vi "QueueDriver.vi"(0 "Queue Name":string, 5 "State & Data":T1, 7 "Array of States & Data":T1[](array[typedef]), 11 "Error in (no error)":errorcluster, 13 "Operations":T2) -> (4 "Dequeued State & Variant":T1, 15 "Error out":errorcluster)   [LabVIEW 2020]
uses:
  Typedef/QueueOperation.ctl
  Typedef/State & Varaint.ctl
panel:
  # "Queue Driver"
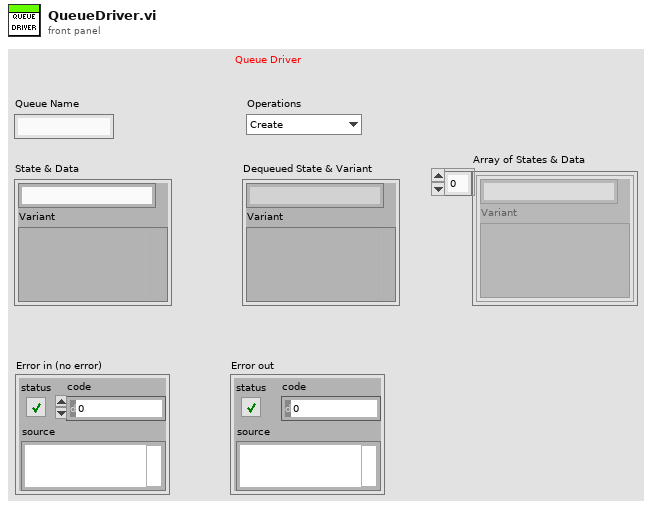
[diagram p1: front panel]
types:
  T1 = typedef "State & Varaint.ctl" = cluster{"State":string, "Variant":variant}
  T2 = typedef "QueueOperation.ctl" = enum16{"Create", "Enqueue 1", "Enqueue N", "Enstack 1", "Enstack N", "Dequeue", "Flush", "Release"}
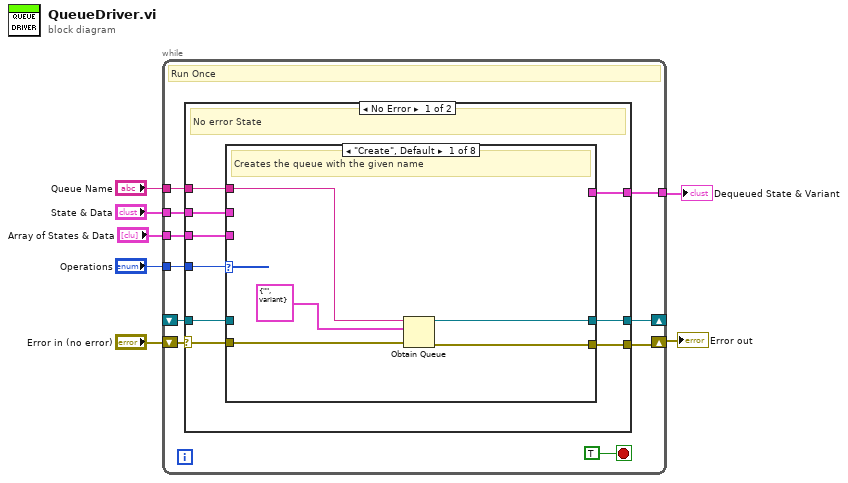
[diagram p0: block diagram]
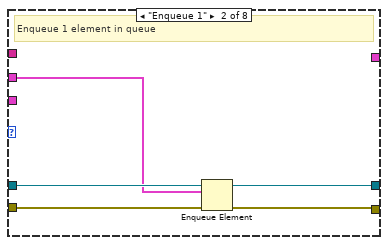
[diagram p2: hidden frame]
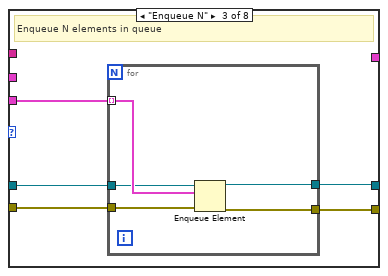
[diagram p3: hidden frame]
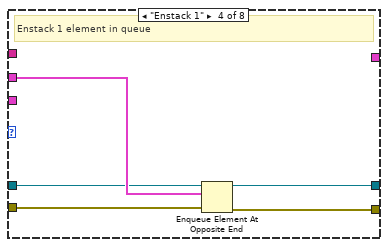
[diagram p4: hidden frame]
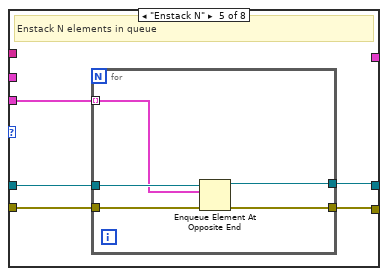
[diagram p5: hidden frame]
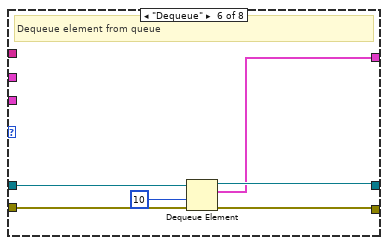
[diagram p6: hidden frame]
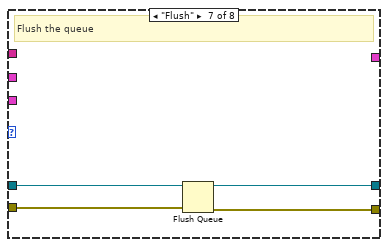
[diagram p7: hidden frame]
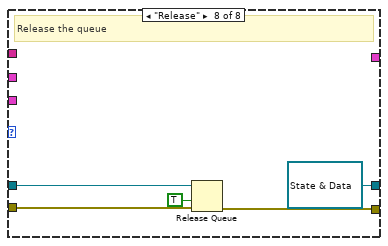
[diagram p8: hidden frame]
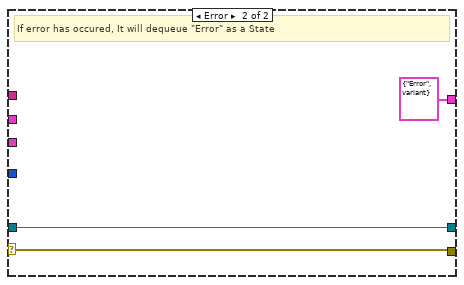
[diagram p9: hidden frame]
diagram:
  n1 = while {
    tunnel: "Operations" -> [w17]
    tunnel: "Queue Name" -> [w14]
    shift-right: [w9] -> _
    shift-left: _ -> [w12]
    tunnel: "State & Data" -> [w11]
    tunnel: "Array of States & Data" -> [w10]
    tunnel: [w8] -> w1
    shift-right: [w13] -> w4
    shift-left: "Error in (no error)" -> [w15]
    stop <- TRUE stop-if-true
    # "Run Once"
    n2 = case shown="No Error" w15 {
      selector: w15 -> [w25 w77]
      tunnel: w17 -> [w26 _]
      tunnel: w14 -> [w24 _]
      tunnel: [w23 w77] -> w13
      tunnel: w12 -> [w22 w78]
      tunnel: w11 -> [w21 _]
      tunnel: w10 -> [w20 _]
      tunnel: [w19 w78] -> w9
      tunnel: [w18 T1 {"State"="Error", "Variant"=variant} ("State & Data")] -> w8
      frame No Error {
        # "No error State"
        n3 = case shown="\"Create\", Default" w26 {
          tunnel: w25 -> [w31 w36 w41 w51 w56 w67 w71 w76]
          tunnel: w24 -> [w30 _ _ _ _ _ _ _]
          tunnel: [w29 w35 w40 w50 w55 w66 w70 w75] -> w23
          tunnel: [w27 w33 w37 w47 w52 w64 w68 refnum<queue> refnum ("queue out")] -> w19
          tunnel: w22 -> [_ w34 w38 w48 w53 w65 w69 w74]
          tunnel: w21 -> [_ w32 _ w49 _ _ _ _]
          tunnel: w20 -> [_ _ w39 _ w54 _ _ _]
          tunnel: [_ _ _ _ _ w63 _ _] -> w18
          frame "Create", Default {
            # "Creates the queue with the given name"
            n4 = Obtain Queue(name (unnamed)=w30, element data type=T1 {"State"="", "Variant"=variant} ("State & Data"), error in (no error)=w31) -> (queue out=w27:refnum<queue>, error out=w29:errorcluster)  [unwired: 2 in, 1 out]
          }
          frame "Enqueue 1" {
            # "Enqueue 1 element in queue"
            n5 = Enqueue Element(queue=w34, element=w32, error in (no error)=w36) -> (queue out=w33:refnum<queue>, error out=w35:errorcluster)  [unwired: 1 in, 1 out]
          }
          frame "Enqueue N" {
            # "Enqueue N elements in queue"
            n6 = for {
              tunnel: w41 -> [w46]
              tunnel: [w45] -> w40
              tunnel: w39 -> [w44] mode=indexing
              tunnel: w38 -> [w43]
              tunnel: [w42] -> w37
              n7 = Enqueue Element(queue=w43, element=w44, error in (no error)=w46) -> (queue out=w42:refnum<queue>, error out=w45:errorcluster)  [unwired: 1 in, 1 out]
            }
          }
          frame "Enstack 1" {
            # "Enstack 1 element in queue"
            n8 = Enqueue Element At Opposite End(queue=w48, element=w49, error in (no error)=w51) -> (queue out=w47:refnum<queue>, error out=w50:errorcluster)  [unwired: 1 in, 1 out]
          }
          frame "Enstack N" {
            # "Enstack N elements in queue"
            n9 = for {
              tunnel: w56 -> [w61]
              tunnel: [w60] -> w55
              tunnel: w54 -> [w57] mode=indexing
              tunnel: w53 -> [w59]
              tunnel: [w58] -> w52
              n10 = Enqueue Element At Opposite End(queue=w59, element=w57, error in (no error)=w61) -> (queue out=w58:refnum<queue>, error out=w60:errorcluster)  [unwired: 1 in, 1 out]
            }
          }
          frame "Dequeue" {
            # "Dequeue element from queue"
            n11 = Dequeue Element(queue=w65, timeout in ms (-1)=10, error in (no error)=w67) -> (queue out=w64:refnum<queue>, element=w63:T1, error out=w66:errorcluster)  [unwired: 1 out]
          }
          frame "Flush" {
            # "Flush the queue"
            n12 = Flush Queue(queue=w69, error in (no error)=w71) -> (queue out=w68:refnum<queue>, error out=w70:errorcluster)  [unwired: 1 out]
          }
          frame "Release" {
            # "Release the queue"
            n13 = Release Queue(queue=w74, force destroy? (F)=TRUE, error in (no error)=w76) -> (error out=w75:errorcluster)  [unwired: 2 out]
          }
        }
      }
      frame Error {
        # "If error has occured, It will dequeue \"Error\" as a State"
      }
    }
  }
  "Error out" <- w4
  "Dequeued State & Variant" <- w1
